vi "Process triangle (partial).vi"(1 "Triangle in":T1) -> (0 "Triangle out":T1)   [LabVIEW 2014]
doc: "This VI must be run after any alteration to the triangles geometry involving scaling and rotation.\nThere is no need to run this VI after applying a translation."
uses:
  Typedefs/Triangle.ctl
  Subroutines/Cross product 3D.vi
  Subroutines/Unit vector.vi
  Subroutines/Dot product.vi
panel:
  # "PN 13/01/2015"
  # "Vertices"
  # "Edges"
  # "Unit normal"
  # "Edge unit normals"
  # "Vertices"
  # "Edges"
  # "Unit normal"
  # "Edge unit normals"
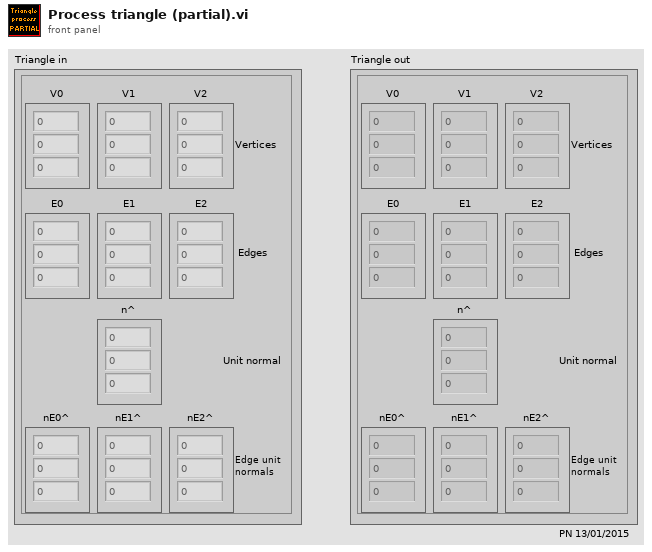
[diagram p1: front panel]
types:
  T1 = typedef "Triangle.ctl" = cluster{"V0":sgl[], "V1":sgl[], "V2":sgl[], "E0":sgl[], "E1":sgl[], "E2":sgl[], "n^":sgl[], "nE0^":sgl[], "nE1^":sgl[], "nE2^":sgl[]}
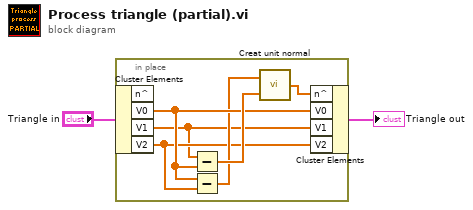
[diagram p0: block diagram]
diagram:
  n1 = in-place {
    n2 = in-place-cluster #1("Triangle in") -> ("V0"=w6:sgl[], "V1"=w3:sgl[], "V2"=w4:sgl[])  [unwired: 1 out]
    n3 = Subtract(x=w3, y=w6) -> (x-y=w7:sgl[])
    n4 = Subtract(x=w6, y=w4) -> (x-y=w5:sgl[])
    n5 = call "Creat unit normal.vi"("E2"=w7, "E1"=w5) -> ("n^ = (E1 x E2) / ||E1 x E2||"=w8:sgl[])
    n6 = in-place-cluster #1("n^"=w8, "V0"=w6, "V1"=w3, "V2"=w4) -> (→"Triangle out":T1)
  }
